vi "Draw Trajectory.vi"(7 "Robot Index":i32, 9 "new picture in":picture, 10 "Trajectory Data":T2(array[cluster]), 11 "Picture in":refnum<vi>) -> (2 "Output Point":T1, 3 "new picture":picture)   [LabVIEW 2019]
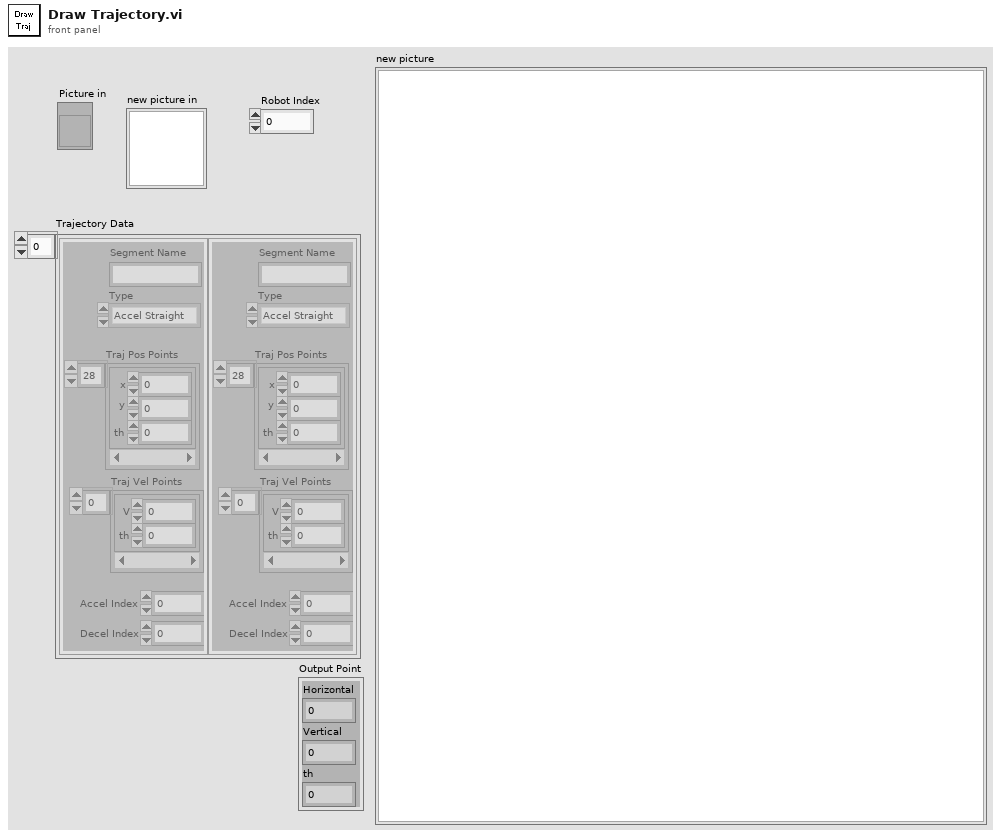
[diagram p1: front panel]
types:
  T1 = cluster{"Horizontal":dbl, "Vertical":dbl, "th":dbl}
  T2 = cluster{"Segment Name":string, "Type":enum16{"Accel Straight", "Const Straight", "Blend", "Circle"}, "Traj Pos Points":cluster{"x":dbl, "y":dbl, "th":dbl}[], "Traj Vel Points":cluster{"V":dbl, "th":dbl}[], "Accel Index":i32, "Decel Index":i32}[]
  T3 = cluster{"Width":u16, "Style":enum32{"Solid", "Dash", "Dot", "DashDot", "DashDotDot"}}
  T4 = typedef "LVPositionTypeDef.ctl" = cluster{"Left":i32, "Top":i32}
  T5 = typedef "LVBoundsTypeDef.ctl" = cluster{"Width":u32, "Height":u32}
  T6 = enum16{"Accel Straight", "Const Straight", "Blend", "Circle"}
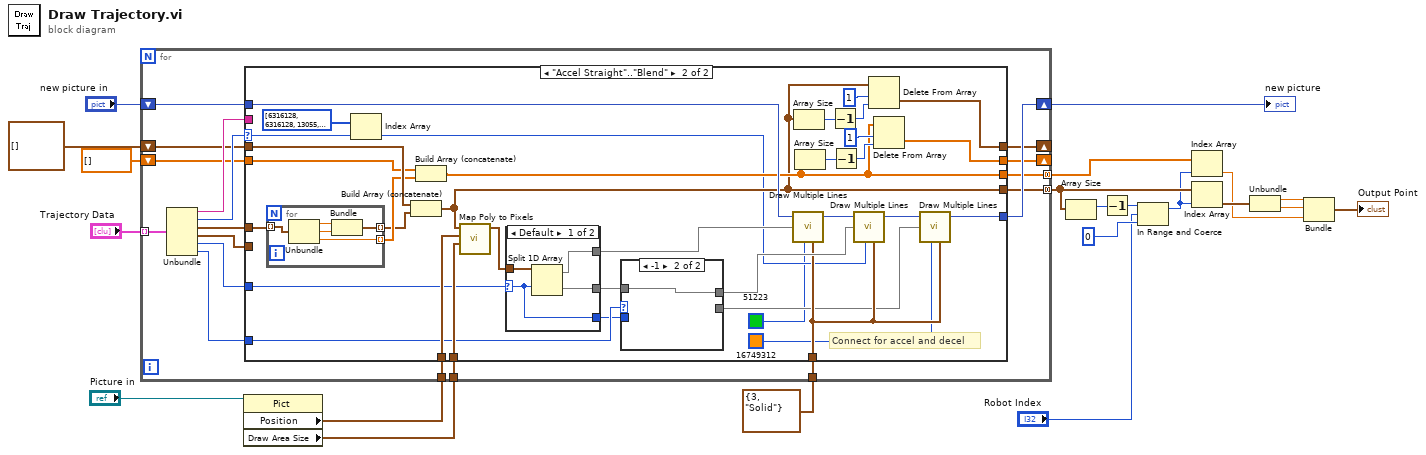
[diagram p0: block diagram]
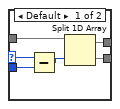
[diagram p3: hidden frame]
diagram:
  n1 = property on="Property Node" class="Pict"(reference="Picture in") -> ("Position"=w16:T4, "Draw Area Size"=w17:T5)  [unwired: 1 in, 2 out]
  n2 = for {
    tunnel: "Trajectory Data" -> [w39] mode=indexing
    shift-right: [w32] -> w15
    shift-left: "new picture in" -> [w31]
    tunnel: T3 {"Width"=3, "Style"=enum."Solid"} ("pen") -> [w35]
    tunnel: w17 -> [w34]
    tunnel: w16 -> [w33]
    tunnel: [w29] -> w8 mode=concatenating
    tunnel: [w28] -> w9 mode=concatenating
    shift-right: [w26] -> _
    shift-left: cluster{"x":dbl, "y":dbl}[] [] -> [w25]
    shift-right: [w24] -> _
    shift-left: dbl[] [] -> [w23]
    n3 = Unbundle(w39) -> ("Segment Name"=w38:string, "Type"=w30:T6, "Traj Pos Points"=w37:cluster{"x":dbl, "y":dbl, "th":dbl}[], "Traj Vel Points"=w36:cluster{"V":dbl, "th":dbl}[], "Accel Index"=w27:i32, "Decel Index"=w22:i32)
    n4 = case shown="\"Accel Straight\"..\"Blend\"" w30 {
      selector: w30 -> [_ w73]
      tunnel: w38 -> [_ _]
      tunnel: w37 -> [_ w77]
      tunnel: w36 -> [_ _]
      tunnel: w35 -> [_ w53]
      tunnel: w34 -> [_ w76]
      tunnel: w33 -> [_ w74]
      tunnel: [w42 w54] -> w32
      tunnel: w31 -> [w42 w75]
      tunnel: [_ w48] -> w29
      tunnel: [_ w62] -> w28
      tunnel: w27 -> [_ w59]
      tunnel: [w41 w67] -> w26
      tunnel: w25 -> [w41 w70]
      tunnel: [w40 w63] -> w24
      tunnel: w23 -> [w40 w60]
      tunnel: w22 -> [_ w58]
      frame Default {
      }
      frame "Accel Straight".."Blend" {
        # "Connect for accel and decel"
        n5 = for {
          tunnel: w77 -> [w94] mode=indexing
          tunnel: [w93] -> w49 mode=indexing
          tunnel: [w90] -> w61 mode=indexing
          n6 = Unbundle(w94) -> ("x"=w92:dbl, "y"=w91:dbl, "th"=w90:dbl)
          n7 = Bundle("x"=w92, "y"=w91) -> (w93:cluster{"x":dbl, "y":dbl})  [unwired: 1 in]
        }
        n8 = Index Array(array=u32[] [6316128, 6316128, 13055, 16771584], index=w73) -> (element=w44:u32)
        n9 = Build Array (concatenate)(w70, w49) -> (w48:cluster{"x":dbl, "y":dbl}[])
        n10 = Build Array (concatenate)(w60, w61) -> (w62:dbl[])
        n11 = call "Map Poly to Pixels.vi"("Draw Area Size"=w76, "Position"=w74, "Coords"=w48) -> ("Coords"=w47:cluster{"Horizontal":dbl, "Vertical":dbl}[])  [unwired: 8 in]
        n12 = case shown="Default" w59 {
          selector: w59 -> [w85 _]
          tunnel: w47 -> [w88 w89]
          tunnel: [w86 _] -> w46
          tunnel: [w87 w89] -> w51
          tunnel: [w85 _] -> w50
          frame Default {
            n13 = Split 1D Array(array=w88, index=w85) -> (first subarray=w86:cluster{"Horizontal":dbl, "Vertical":dbl}[], second subarray=w87:cluster{"Horizontal":dbl, "Vertical":dbl}[])
          }
          frame -1 {
          }
        }
        n14 = case shown="-1" w58 {
          selector: w58 -> [w80 _]
          tunnel: w51 -> [w83 w84]
          tunnel: [w82 w84] -> w56
          tunnel: [w81 _] -> w52
          tunnel: w50 -> [w79 _]
          frame Default {
            n15 = Subtract(x=w80, y=w79) -> (x-y=w78:i32)
            n16 = Split 1D Array(array=w83, index=w78) -> (first subarray=w82:cluster{"Horizontal":dbl, "Vertical":dbl}[], second subarray=w81:cluster{"Horizontal":dbl, "Vertical":dbl}[])
          }
          frame -1 {
          }
        }
        n17 = call <vilib>:"Draw Multiple Lines.vi"("picture"=w75, "line endpoints"=w46, "color(black)"=u32 51223, "pen"=w53) -> ("new picture"=w57:picture)  [unwired: 5 in]
        n18 = Array Size(array=w48) -> (size(s)=w71:i32)
        n19 = Array Size(array=w62) -> (size(s)=w64:i32)
        n20 = Decrement(x=w71) -> (x-1=w68:i32)
        n21 = Decrement(x=w64) -> (x-1=w66:i32)
        n22 = call <vilib>:"Draw Multiple Lines.vi"("picture"=w57, "line endpoints"=w56, "color(black)"=w44, "pen"=w53) -> ("new picture"=w55:picture)  [unwired: 5 in]
        n23 = Delete From Array(array=w48, length=1, index=w68) -> (deleted portion=w67:cluster{"x":dbl, "y":dbl}[])  [unwired: 1 out]
        n24 = Delete From Array(array=w62, length=1, index=w66) -> (deleted portion=w63:dbl[])  [unwired: 1 out]
        n25 = call <vilib>:"Draw Multiple Lines.vi"("picture"=w55, "line endpoints"=w52, "color(black)"=u32 16749312, "pen"=w53) -> ("new picture"=w54:picture)  [unwired: 5 in]
      }
    }
  }
  "new picture" <- w15
  n26 = Array Size(array=w8) -> (size(s)=w7:i32)
  n27 = Decrement(x=w7) -> (x-1=w6:i32)
  n28 = In Range and Coerce(upper limit=w6, x="Robot Index", lower limit=u16 0 ("Width")) -> (coerced(x)=w3:i32)  [unwired: 1 out]
  n29 = Index Array(array=w9, index=w3) -> (element=w11:dbl)
  n30 = Index Array(array=w8, index=w3) -> (element=w14:cluster{"x":dbl, "y":dbl})
  n31 = Unbundle(w14) -> ("x"=w13:dbl, "y"=w12:dbl)
  n32 = Bundle("x"=w13, "y"=w12, "th"=w11) -> (→"Output Point":cluster{"x":dbl, "y":dbl, "th":dbl})  [unwired: 1 in]
